vi "Alicat cluster to waveform.vi"(1 "Data Cluster in":T2, 2 "Measurement Units in":T1) -> (0 "Array":waveform(dbl)[](array[waveform]))   [LabVIEW 2018]
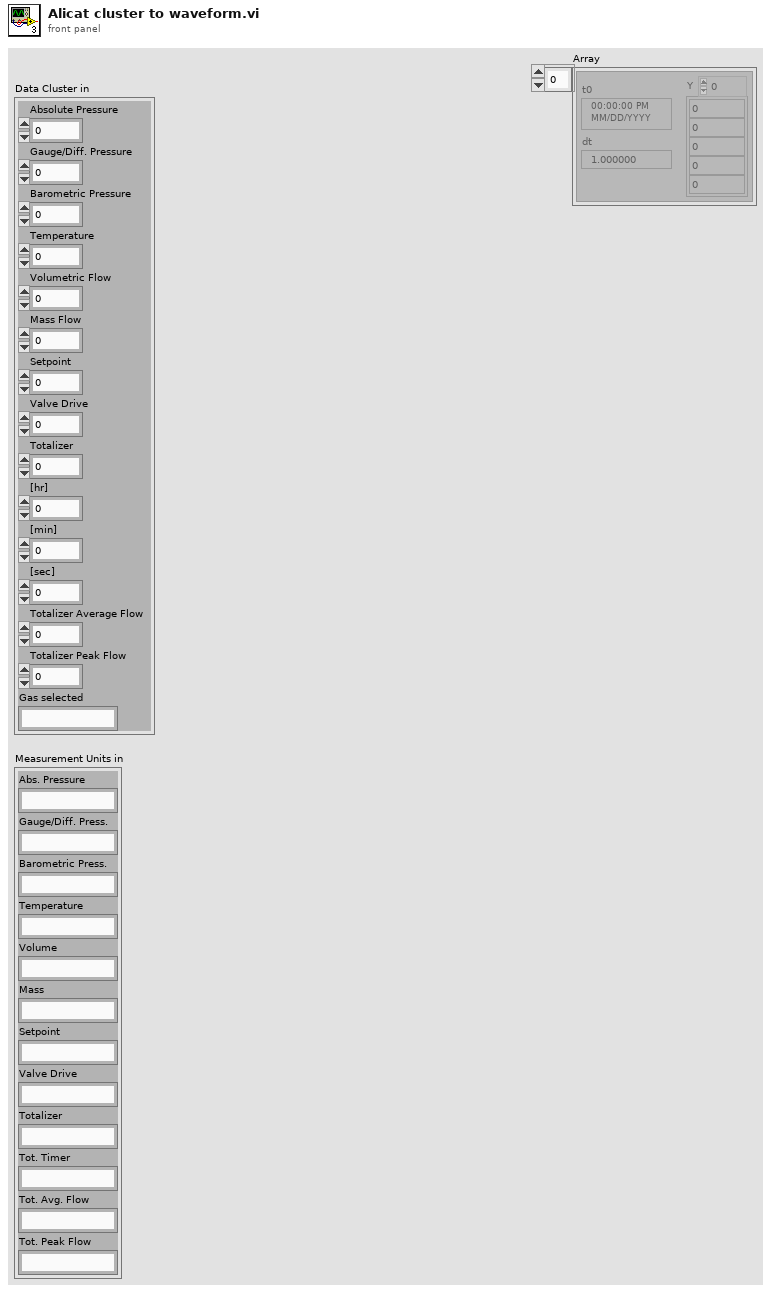
[diagram p1: front panel]
types:
  T1 = cluster{"Abs. Pressure":string, "Gauge/Diff. Press.":string, "Barometric Press.":string, "Temperature":string, "Volume":string, "Mass":string, "Setpoint":string, "Valve Drive":string, "Totalizer":string, "Tot. Timer":string, "Tot. Avg. Flow":string, "Tot. Peak Flow":string}
  T2 = cluster{"Absolute Pressure":dbl, "Gauge/Diff. Pressure":dbl, "Barometric Pressure":dbl, "Temperature":dbl, "Volumetric Flow":dbl, "Mass Flow":dbl, "Setpoint":dbl, "Valve Drive":dbl, "Totalizer":dbl, "[hr]":dbl, "[min]":dbl, "[sec]":dbl, "Totalizer Average Flow":dbl, "Totalizer Peak Flow":dbl, "Gas selected":string}
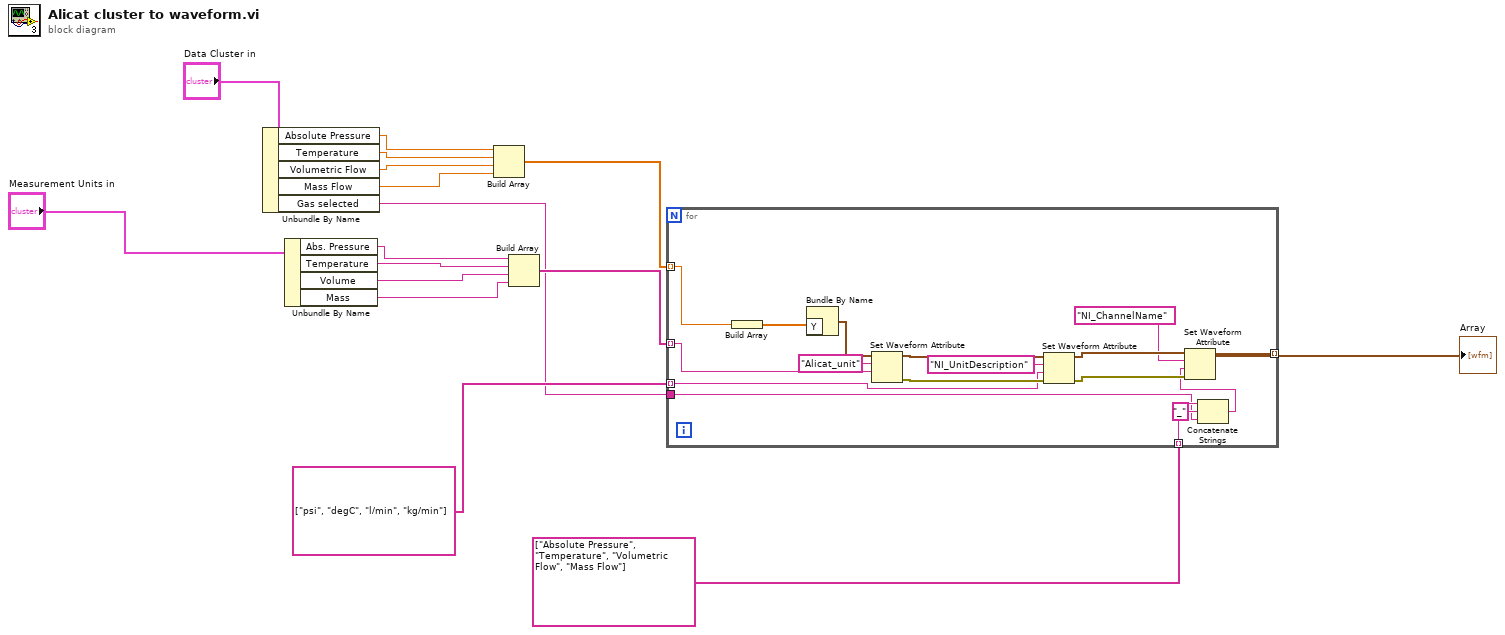
[diagram p0: block diagram]
diagram:
  n1 = Unbundle By Name("Data Cluster in") -> ("Absolute Pressure"=w14:dbl, "Temperature"=w13:dbl, "Volumetric Flow"=w12:dbl, "Mass Flow"=w11:dbl, "Gas selected"=w1:string)
  n2 = Unbundle By Name("Measurement Units in") -> ("Abs. Pressure"=w10:string, "Temperature"=w9:string, "Volume"=w8:string, "Mass"=w7:string)
  n3 = Build Array(w14, w13, w12, w11) -> (w4:dbl[])
  n4 = Build Array(w10, w9, w8, w7) -> (w5:string[])
  n5 = for {
    tunnel: string[] ["psi", "degC", "l/min", "kg/min"] -> [w25] mode=indexing
    tunnel: w5 -> [w30] mode=indexing
    tunnel: w4 -> [w33] mode=indexing
    tunnel: [w23] -> w3 mode=indexing
    tunnel: string[] ["Absolute Pressure", "Temperature", "Volumetric Flow", "Mass Flow"] -> [w20] mode=indexing
    tunnel: w1 -> [w18]
    n6 = Build Array(w33) -> (w32:dbl[])
    n7 = Bundle By Name("Y"=w32) -> (w31:waveform(dbl))  [unwired: 1 in]
    n8 = Set Waveform Attribute(5:w30, 6:"Alicat_unit" ("name"), 7:w31) -> (0:w27:errorcluster, 3:w28:waveform(dbl))  [unwired: 1 in, 1 out]
    n9 = Set Waveform Attribute(4:w27, 5:w25, 6:"NI_UnitDescription" ("name"), 7:w28) -> (0:w22:errorcluster, 3:w24:waveform(dbl))  [unwired: 1 out]
    n10 = Concatenate Strings(w20, "_" ("string"), w18) -> (w17:string)
    n11 = Set Waveform Attribute(4:w22, 5:w17, 6:"NI_ChannelName" ("name"), 7:w24) -> (3:w23:waveform(dbl))  [unwired: 2 out]
  }
  "Array" <- w3
